vi "PH_Beamline.PC _MAInjectBox.vi"(0 "i ref in":refnum<vi>, 3 "Value":i32, 5 "error in (no error)":errorcluster) -> (14 "i ref out":refnum<vi>, 19 "error out":errorcluster)   [LabVIEW 2009, in "PH_Beamline.lvlib"]
doc: "This VI writes the incoming information for the MA injection box state to the related GUI element and to own attributes."
uses:
  PH_Beamline.lvlib
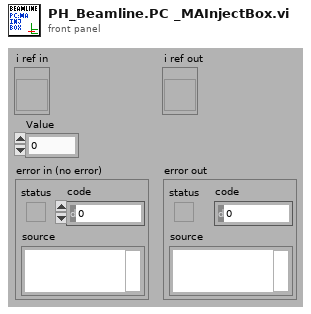
[diagram p1: front panel]
types:
  T1 = typedef "PH_Beamline.lvlib/PH_Beamline.i attribute.ctl" = cluster{"GUI Refs":cluster{"Delete":refnum<vi>, "BL ok":refnum<vi>, "PA ok":refnum<vi>, "MA ok":refnum<vi>, "fs FE ok":refnum<vi>, "ns FE ok":refnum<vi>, "PA ED ok":refnum<vi>, "MAS ok":refnum<vi>, "Booster ok":refnum<vi>, "Mirrortower ok":refnum<vi>, "In.-Box ok":refnum<vi>, "Compressor ok":refnum<vi>, "Experiment LB ok":refnum<vi>, "Experiment LL ok":refnum<vi>, "PHELIX_Beckhoff_Watchdog":refnum<vi>, "Shutters closed":refnum<vi>}, "Beamline State":cluster{"Subsystems":cluster{"PA":bool, "MA":bool, "ns FE":bool, "fs FE":bool, "PA ED":bool, "In.-Box":bool, "MAS":bool, "Booster":bool, "Mirrortower":bool, "Compressor":bool, "Experiment LB":bool, "Experiment LL":bool}, "State":bool}, "Remote Controlled by":string, "R2S ID":i32, "Refs BL MA":refnum<vi>[], "Refs Motion":refnum<vi>[], "Refs Cams":refnum<vi>[], "Refs Ops":refnum<vi>[], "State BBs":T2[], "Refs BBs":refnum<vi>[], "State Switches":T2[], "Refs Switches":refnum<vi>[], "Refs Vac":refnum<vi>[], "Vacua":cluster{"Instance":string, "Channelname":string, "Limit":dbl, "Curr Value":dbl, "in range":bool}[], "Refs BL MA-IB":refnum<vi>[], "Refs BL fs":refnum<vi>[], "Refs BL PA ED":refnum<vi>[], "Refs BL MAS":refnum<vi>[], "Refs Powermeter":refnum<vi>[], "Refs O2":refnum<vi>[], "O2 Inspection":cluster{"Concentration":dbl, "State":T2}[], "Refs BL Boo":refnum<vi>[], "Refs BL ns":refnum<vi>[], "Refs BL Mirrortower":refnum<vi>[], "Refs BL Compressor":refnum<vi>[], "Refs BL Exp LB":refnum<vi>[], "Refs 6P Switches":refnum<vi>[], "State 6P Switches":T2[], "Radiation Safety":cluster{"Exp Laserbay":cluster{"Ref Op Mode":refnum<vi>, "Ref Laserbay evacuated":refnum<vi>, "Tagname LB evacuated":string, "Shot Mode":T3, "Laserbay evacuated?":i32, "Tagname HV room locked":string, "HV room locked?":i32, "Ref HV room locked":refnum<vi>, "Tagname bridged?":string, "Ref Bridge":refnum<vi>, "I<1E18W/cm²":bool}, "Exp Laserlab":cluster{"Ref Op Mode":refnum<vi>, "Ref Laserlab evacuated":refnum<vi>, "Tagname LL evacuated":string, "Shot Mode":T3, "Laserlab evacuated?":i32, "Tagname bridged?":string, "Ref Bridge":refnum<vi>, "I<1E18W/cm²":bool}}, "Refs Switch and Motion":refnum<vi>[], "State Switch and Motion":T2[], "GUI manager Path":string, "Refs BL LL":refnum<vi>[], "Refs Switch GUI":refnum<vi>[], "State Switch GUIs":bool[], "Refs Spectrometer":refnum<vi>[], "PP Igni Heating GUI Refs":refnum<vi>[], "PP Igni Heating Tagnames ":string[], "Refs local GUIs":refnum<vi>[], "Refs BL PA":cluster{"undelayed Line before Shutter":refnum<vi>[], "undelayed Line after Shutter":refnum<vi>[], "before Bypass":refnum<vi>[], "delayed Line before Shutter":refnum<vi>[], "delayed Line after Shutter":refnum<vi>[], "before Shutter Input":refnum<vi>[], "after Shutter Input":refnum<vi>[], "Bypass":refnum<vi>[], "before Shutter Exit":refnum<vi>[], "after Shutter Exit":refnum<vi>[], "to MA":refnum<vi>[], "to Lab":refnum<vi>[]}, "Refs SSACs":refnum<vi>[], "Service ID":cluster{"YLF_BL_Status":i32, "fs_BL_Status":i32, "fs_YLF_BL_Status":i32, "ns_BL_Status":i32, "PA_Input_BL_Status":i32, "PA_UnDelay_BL_Status":i32, "PA_Delay_BL_Status":i32, "PA_BL_Status":i32, "PA_Bypass_BL_Status":i32, "PA_Exit_BL_Status":i32, "PA_LL_BL_Status":i32, "LL_BL_Status":i32, "PA_MA_BL_Status":i32, "MA_Exit_BL_Status":i32, "MA_Z6_BL_Status":i32, "Z6_BL_Status":i32, "MA_LB_BL_Status":i32, "LB_TB2_BL_Status":i32, "PA_before_Bypass_BL_Status":i32, "LB_TB3_BL_Status":i32}, "BL":cluster{"YLF_BL_Status":i32, "fs_BL_Status":i32, "fs_YLF_BL_Status":i32, "ns_BL_Status":i32, "PA_Input_BL_Status":i32, "PA_UnDelay_BL_Status":i32, "PA_Delay_BL_Status":i32, "PA_BL_Status":i32, "PA_Bypass_BL_Status":i32, "PA_Exit_BL_Status":i32, "PA_LL_BL_Status":i32, "LL_BL_Status":i32, "PA_MA_BL_Status":i32, "MA_Exit_BL_Status":i32, "MA_Z6_BL_Status":i32, "Z6_BL_Status":i32, "MA_LB_BL_Status":i32, "LB_TB2_BL_Status":i32, "PA_before_Bypass_BL_Status":i32, "LB_TB3_BL_Status":i32}, "Refs Existance Booleans":refnum<vi>[], "Refs free Motion GUIs":refnum<vi>[], "Refs Crosshairs":refnum<vi>[]}
  T2 = typedef "Status.ctl" = i16
  T3 = typedef "Operation Mode.ctl" = i32
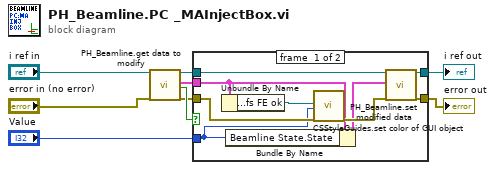
[diagram p0: block diagram]
diagram:
  n1 = call "PH_Beamline.get data to modify.vi"("i ref in"="i ref in", "error in (no error)"="error in (no error)") -> ("i ref out"=w4:refnum<vi>, "i attribute"=w8:T1, "timed out"=w9:bool, "error out"=w6:errorcluster)  [unwired: 14 in]
  n2 = case shown="False" w9 {
    tunnel: w4 -> [w18 w20]
    tunnel: [w17 w20] -> w5
    tunnel: w6 -> [w15 w19]
    tunnel: [w16 w19] -> w7
    tunnel: w8 -> [w13 _]
    tunnel: "Value" -> [w10 _]
    frame #0 {
      n3 = Unbundle By Name(w13) -> ("GUI Refs.fs FE ok"=w11:refnum<vi>)
      n4 = Bundle By Name(cluster=w13, "Beamline State.State"=w10) -> (w12:T1)
      n5 = call "CSStyleGuides.set color of GUI object.vi"("GUI object Ref"=w11, "State"=w10, "error in (no error)"=w15) -> ("error out"=w14:errorcluster)  [unwired: 16 in]
      n6 = call "PH_Beamline.set modified data.vi"("i ref in"=w18, "i attribute"=w12, "error in (no error)"=w14) -> ("i ref out"=w17:refnum<vi>, "error out"=w16:errorcluster)  [unwired: 15 in]
    }
    frame #1 {
    }
  }
  "error out" <- w7
  "i ref out" <- w5
